vi "BiColor Maskv1.vi"(1 "Second Mask":T1, 2 "First Mask":T1, 3 "Rectangle":i32[](array[numeric])) -> (0 "Image Dst Out":T1)   [LabVIEW 2013]
uses:
  <vilib>/vision/Image Controls.llb/IMAQ Image.ctl
  <vilib>/vision/NI_Vision_Development_Module.lvlib
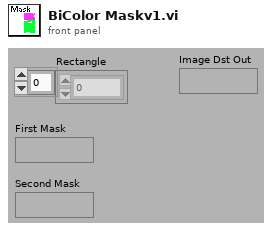
[diagram p1: front panel]
types:
  T1 = typedef "IMAQ Image.ctl" = refnum<image>
  T2 = typedef "Image Type" = u32
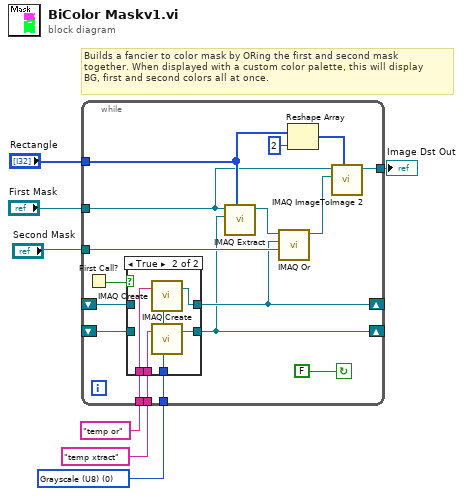
[diagram p0: block diagram]
diagram:
  w2 = T2 0 items=["Grayscale (U8)", "Grayscale (I16)", "Grayscale (SGL)", "Complex (CSG)", "RGB (U32)", "HSL (U32)", "RGB (U64)", "Grayscale (U16)"] ("Image Type")
  # "Builds a fancier to color mask by ORing the first and second mask\ntogether. When displayed with a custom color palette, this will display\nBG, first and second colors all at once."
  n1 = while {
    tunnel: [w24] -> w7
    tunnel: "Rectangle" -> [w21]
    tunnel: "First Mask" -> [w20]
    tunnel: "Second Mask" -> [w17]
    shift-right: [w14] -> _
    shift-left: _ -> [w15]
    tunnel: "temp or" -> [w13]
    tunnel: w2 -> [w12]
    tunnel: "temp xtract" -> [w10]
    shift-right: [w8] -> _
    shift-left: _ -> [w9]
    stop <- FALSE continue-if-true
    n2 = First Call?() -> (First Call?: T/F=w16:bool)
    n3 = case shown="True" w16 {
      tunnel: w15 -> [w26 _]
      tunnel: [w26 w31] -> w14
      tunnel: w13 -> [_ w30]
      tunnel: w12 -> [_ w29]
      tunnel: w10 -> [_ w28]
      tunnel: [w25 w27] -> w8
      tunnel: w9 -> [w25 _]
      frame False {
      }
      frame True {
        n4 = call "IMAQ Create"("Image Name"=w30, "Image Type"=w29) -> ("New Image"=w31:T1)  [unwired: 2 in, 2 out]
        n5 = call "IMAQ Create"("Image Name"=w28, "Image Type"=w29) -> ("New Image"=w27:T1)  [unwired: 2 in, 2 out]
      }
    }
    n6 = call "IMAQ Extract"("Optional Rectangle"=w21, "Image Dst"=w8, "Image Src"=w20) -> ("Image Dst Out"=w18:T1)  [unwired: 3 in, 5 out]
    n7 = call "IMAQ Or"("Image Src B"=w17, "Image Dst"=w14, "Image Src A"=w18) -> ("Image Dst Out"=w19:T1)  [unwired: 3 in, 5 out]
    n8 = Reshape Array(w21, 2 ("dimension size")) -> (w23:i32[])
    n9 = call "IMAQ ImageToImage 2"("Offset Left/Top"=w23, "Image Src (Small)"=w19, "Image Src (Large)"=w20) -> ("Image Dst Out"=w24:T1)  [unwired: 3 in, 5 out]
  }
  "Image Dst Out" <- w7
